vi "Limelight Targetting (SubVI).vi"() -> (0 "targetObtained":bool, 3 "Output cluster":T1)   [LabVIEW 2020]
uses:
  <vilib>/Rock Robotics/Network Tables/NT Read Number.vi
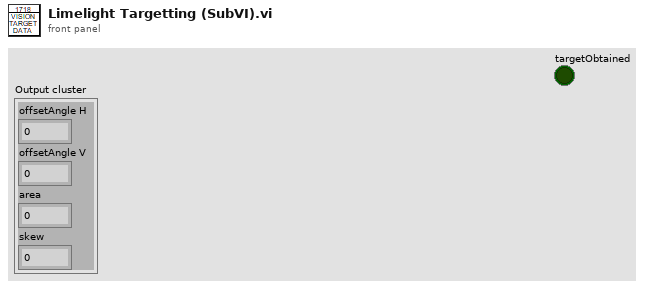
[diagram p1: front panel]
types:
  T1 = cluster{"offsetAngle H":dbl, "offsetAngle V":dbl, "area":dbl, "skew":dbl}
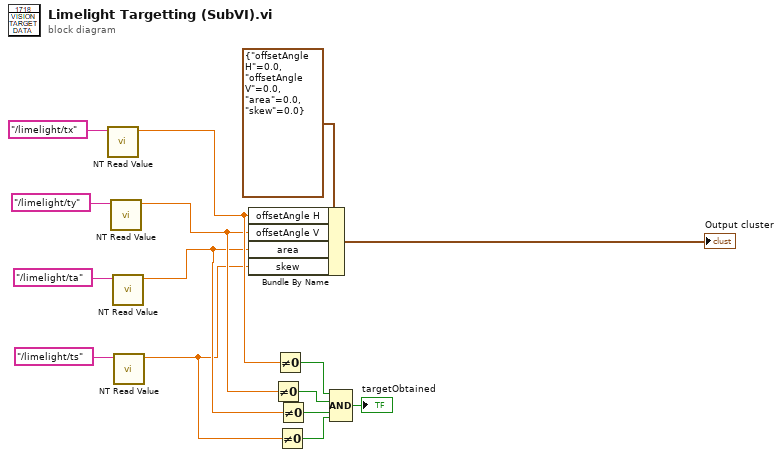
[diagram p0: block diagram]
diagram:
  n1 = call-poly <vilib>:"NT Read Value.vi"("Name"="/limelight/tx") -> ("Numeric"=w9:dbl)  [unwired: 9 in, 1 out]
  n2 = call-poly <vilib>:"NT Read Value.vi"("Name"="/limelight/ty") -> ("Numeric"=w8:dbl)  [unwired: 9 in, 1 out]
  n3 = call-poly <vilib>:"NT Read Value.vi"("Name"="/limelight/ta") -> ("Numeric"=w7:dbl)  [unwired: 9 in, 1 out]
  n4 = call-poly <vilib>:"NT Read Value.vi"("Name"="/limelight/ts") -> ("Numeric"=w6:dbl)  [unwired: 9 in, 1 out]
  n5 = Bundle By Name(cluster=T1 {"offsetAngle H"=0.0, "offsetAngle V"=0.0, "area"=0.0, "skew"=0.0} ("input cluster"), "offsetAngle H"=w9, "offsetAngle V"=w8, "area"=w7, "skew"=w6) -> (→"Output cluster":T1)
  n6 = Not Equal To 0?(x=w8) -> (x != 0?=w4:bool)
  n7 = Not Equal To 0?(x=w9) -> (x != 0?=w5:bool)
  n8 = Not Equal To 0?(x=w6) -> (x != 0?=w2:bool)
  n9 = Not Equal To 0?(x=w7) -> (x != 0?=w3:bool)
  n10 = Compound Arithmetic op=AND(w5, w4, w3, w2) -> (→"targetObtained":bool)
